vi "Run Service.vi"() -> ()   [LabVIEW 2019, in "Generated_server.lvlib"]
uses:
  Generated_server.lvlib
  <vilib>/gRPC/LabVIEW gRPC Servicer/Servicer/Servicer.lvclass/Servicer.ctl
  <vilib>/gRPC/LabVIEW gRPC Servicer/Servicer/Servicer.lvclass
  RPC Service/RouteGuide/RouteGuide.lvclass
panel:
  in  "Async [T] / Sync [F]":bool
  out "Listening Port":i32
  in  "Stop":bool
  in  "Server Address":string="localhost:50051"
  in  "Server Certificate File (.crt)":path
  in  "Server Key File (.key)":path
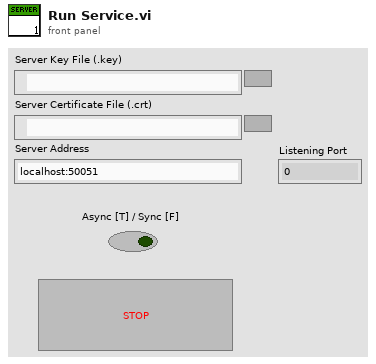
[diagram p1: front panel]
types:
  T1 = typedef "grpc-lvsupport-release.lvlib/grpcId.ctl" = u64
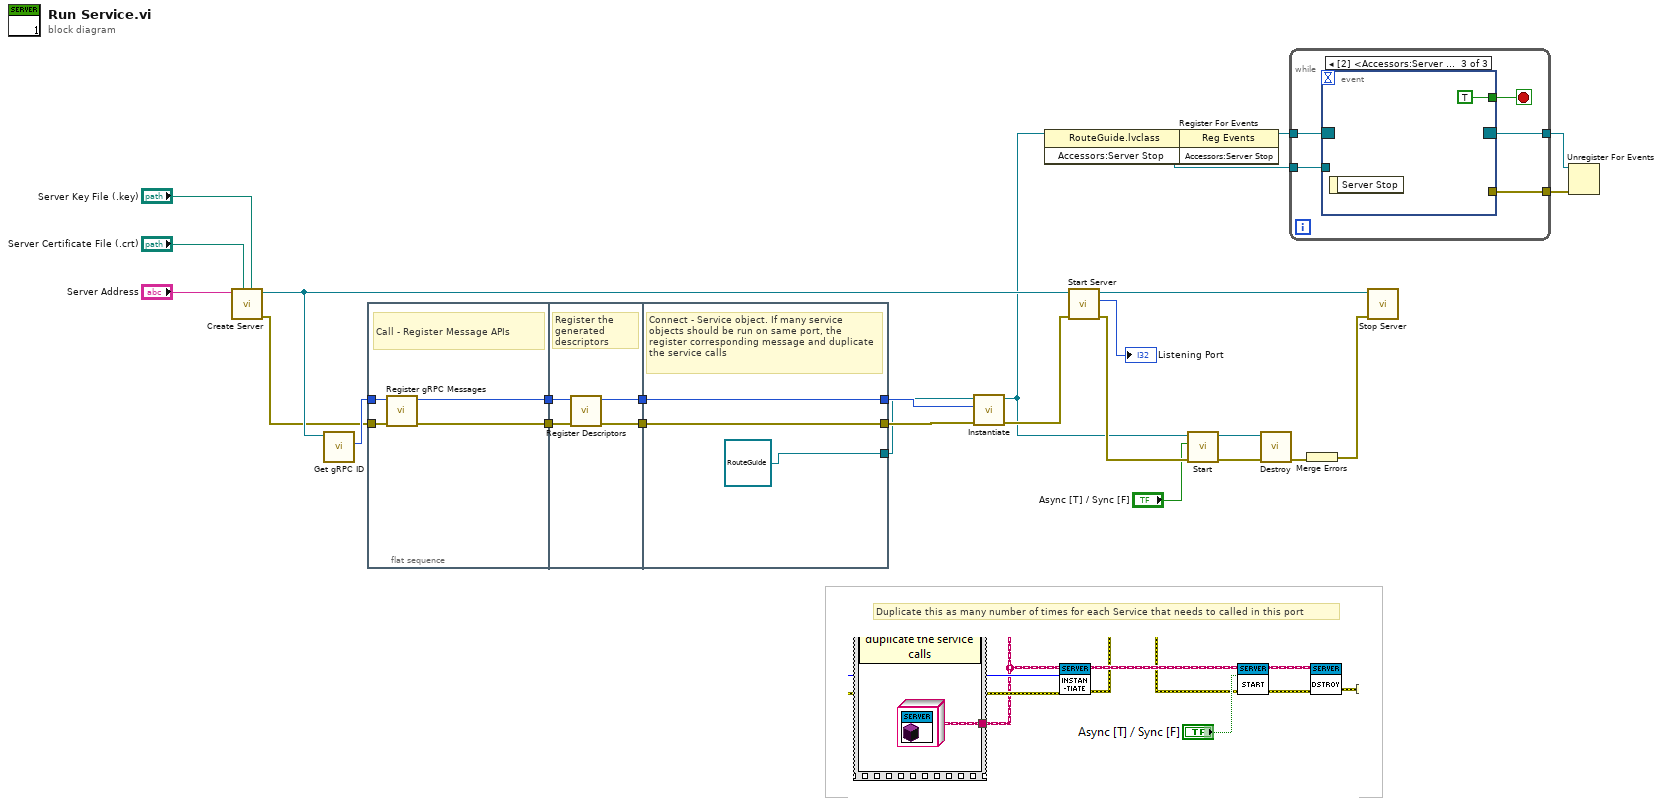
[diagram p0: block diagram]
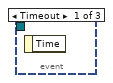
[diagram p2: hidden frame]
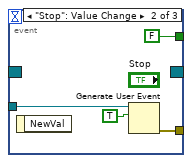
[diagram p3: hidden frame]
diagram:
  # "Duplicate this as many number of times for each Service that needs to called in this port"
  n1 = call <vilib>:"Create Server.vi"("Server Key File (.key)"="Server Key File (.key)", "Server Certificate File (.crt)"="Server Certificate File (.crt)", "Server Address"="Server Address") -> ("error out"=w14:errorcluster, "gRPC Server out"=w21:refnum<class "Servicer.lvclass">)  [unwired: 7 in]
  n2 = call <vilib>:"Get gRPC ID.vi"("OOP Server in"=w21) -> ("gRPC ID"=w15:T1)  [unwired: 9 in, 1 out]
  n3 = flat-sequence {
    tunnel: w15 -> [w30]
    tunnel: w14 -> [w32]
    tunnel: [w31] -> w5
    tunnel: [w29] -> w4
    tunnel: w5 -> [w35]
    tunnel: w4 -> [w36]
    tunnel: [w33] -> w3
    tunnel: [w34] -> w2
    tunnel: [w38] -> w12
    tunnel: [w39] -> w13
    tunnel: w3 -> [w39]
    tunnel: w2 -> [w38]
    tunnel: [refnum<class "RouteGuide.lvclass"> refnum ("Generated_server.lvlib:RouteGuide.lvclass")] -> w1
    frame #0 {
      # "Call - Register Message APIs"
      n4 = call "Register gRPC Messages.vi"("error in (no error)"=w32, "gRPC ID"=w30) -> ("error out"=w31:errorcluster, "gRPC ID Out"=w29:T1)  [unwired: 8 in]
    }
    frame #1 {
      # "Register the generated descriptors"
      n5 = call "Register Descriptors.vi"("error in (no error)"=w35, "gRPC ID"=w36) -> ("error out"=w33:errorcluster, "gRPC ID Out"=w34:T1)  [unwired: 8 in]
    }
    frame #2 {
      # "Connect - Service object. If many service objects should be run on same port, the register corresponding message and duplicate the service calls"
    }
  }
  n6 = call-dynamic "Instantiate.vi"("error in"=w13, "gRPCid"=w12, "iService"=w1) -> ("error out"=w19:errorcluster, "iService"=w7:refnum<class "RouteGuide.lvclass">)  [unwired: 7 in]
  n7 = property class="RouteGuide.lvclass"(reference=w7) -> (error out=w20:errorcluster, "Accessors:Server Stop"=w6:refnum<user-event>)  [unwired: 1 in, 1 out]
  n8 = call <vilib>:"Start Server.vi"("error in"=w19, "gRPC Server in"=w21) -> ("error out"=w11:errorcluster, "Listening Port"=→"Listening Port":i32, "gRPC Server out"=w28:refnum<class "Servicer.lvclass">)  [unwired: 7 in]
  n9 = register-events(error in=w20, w6) -> (reference out=w24:refnum<event-registration>)  [unwired: 1 in, 1 out]
  n10 = call-dynamic "Start.vi"("error in"=w11, "ASync [T]"="Async [T] / Sync [F]", "iService in"=w7) -> ("error out"=w10:errorcluster, "iService out"=w9:refnum<class "RouteGuide.lvclass">)  [unwired: 7 in]
  n11 = call-dynamic "Destroy.vi"("error in (no error)"=w10, "SignalGeneratorService in"=w9) -> ("error out"=w18:errorcluster)  [unwired: 8 in, 1 out]
  n12 = while {
    tunnel: w24 -> [w44]
    tunnel: [w42] -> w23
    tunnel: [w40] -> w16
    tunnel: w6 -> [w41]
    stop <- w43 stop-if-true
    n13 = event shown="[2] <Accessors:Server Stop>: User Event" {
      selector: w44 -> [_ _ _]
      dyn-events: [_ _ _] -> w42
      timeout: _ -> [_ _ _]
      tunnel: [_ FALSE TRUE] -> w43
      tunnel: w41 -> [_ w47 _]
      tunnel: [_ w45 _] -> w40
      event Timeout {
        n14 = event-data() -> ()  [unwired: 1 in, 1 out]
      }
      event "Stop": Value Change {
        n15 = event-data() -> ()  [unwired: 1 in, 1 out]
        n16 = Generate User Event(user event=w47, event data cluster=TRUE ("event data")) -> (error out=w45:errorcluster)  [unwired: 2 in, 1 out]
      }
      event User Event {
        n17 = event-data() -> ()  [unwired: 1 in, 1 out]
      }
    }
  }
  n18 = Merge Errors(w18) -> (w17:errorcluster)
  n19 = call <vilib>:"Stop Server.vi"("error in"=w17, "gRPC Server in"=w28) -> ()  [unwired: 9 in, 1 out]
  n20 = Unregister For Events(event registration refnum=w23, error in=w16) -> ()  [unwired: 1 out]
